vi "Chart_Formula_Manual_Incremental.vi"(7 "error in (no error)":errorcluster, 9 "Max Voltage":dbl, 10 "Min Voltage":dbl) -> ()   [LabVIEW 2020]
uses:
  Global 1.vi
panel:
  out "INDEX TI - 5th":i32
  out "ADDER TI - 5th":dbl
  out "INDEX TI - 4th":i32
  out "ADDER TI - 4th":dbl
  out "INDEX TI - 3rd":i32
  out "ADDER TI - 3rd":dbl
  out "INDEX TI - 2nd":i32
  out "ADDER TI - 2nd":dbl
  out "INDEX TI - 1st":i32
  out "size(s)":i32
  out "ADDER TI - 1st":dbl
  out "Array TI - 5th":dbl[](array[numeric])
  out "Array TI - 4th":dbl[](array[numeric])
  out "Array TI - 3rd":dbl[](array[numeric])
  out "Array TI - 2nd":dbl[](array[numeric])
  out "Array TI - 1st":dbl[](array[numeric])
  out "Chosen Max Voltage":dbl
  out "Chosen Min Voltage":dbl
  out "error out":errorcluster
  in  "CONFIRM CONDITION?":bool
  in  "Use 5th Threshold & Incremental ?":bool
  in  "Use 4th Threshold & Incremental ?":bool
  in  "Use 3rd Threshold & Incremental ?":bool
  in  "Use 2nd Threshold & Incremental ?":bool
  in  "Use 1st Threshold & Incremental ?":bool
  in  "Incremental 5":dbl
  in  "Threshold 5":dbl
  in  "Incremental 4":dbl
  in  "Threshold 4":dbl
  in  "Incremental 3":dbl
  in  "Threshold 3":dbl
  in  "Incremental 2":dbl
  in  "Threshold 2":dbl
  in  "Incremental 1":dbl
  in  "Threshold 1":dbl
  out "Array Result":dbl[](array[numeric])
  # "Manual Incremental : Increment at Threshold"
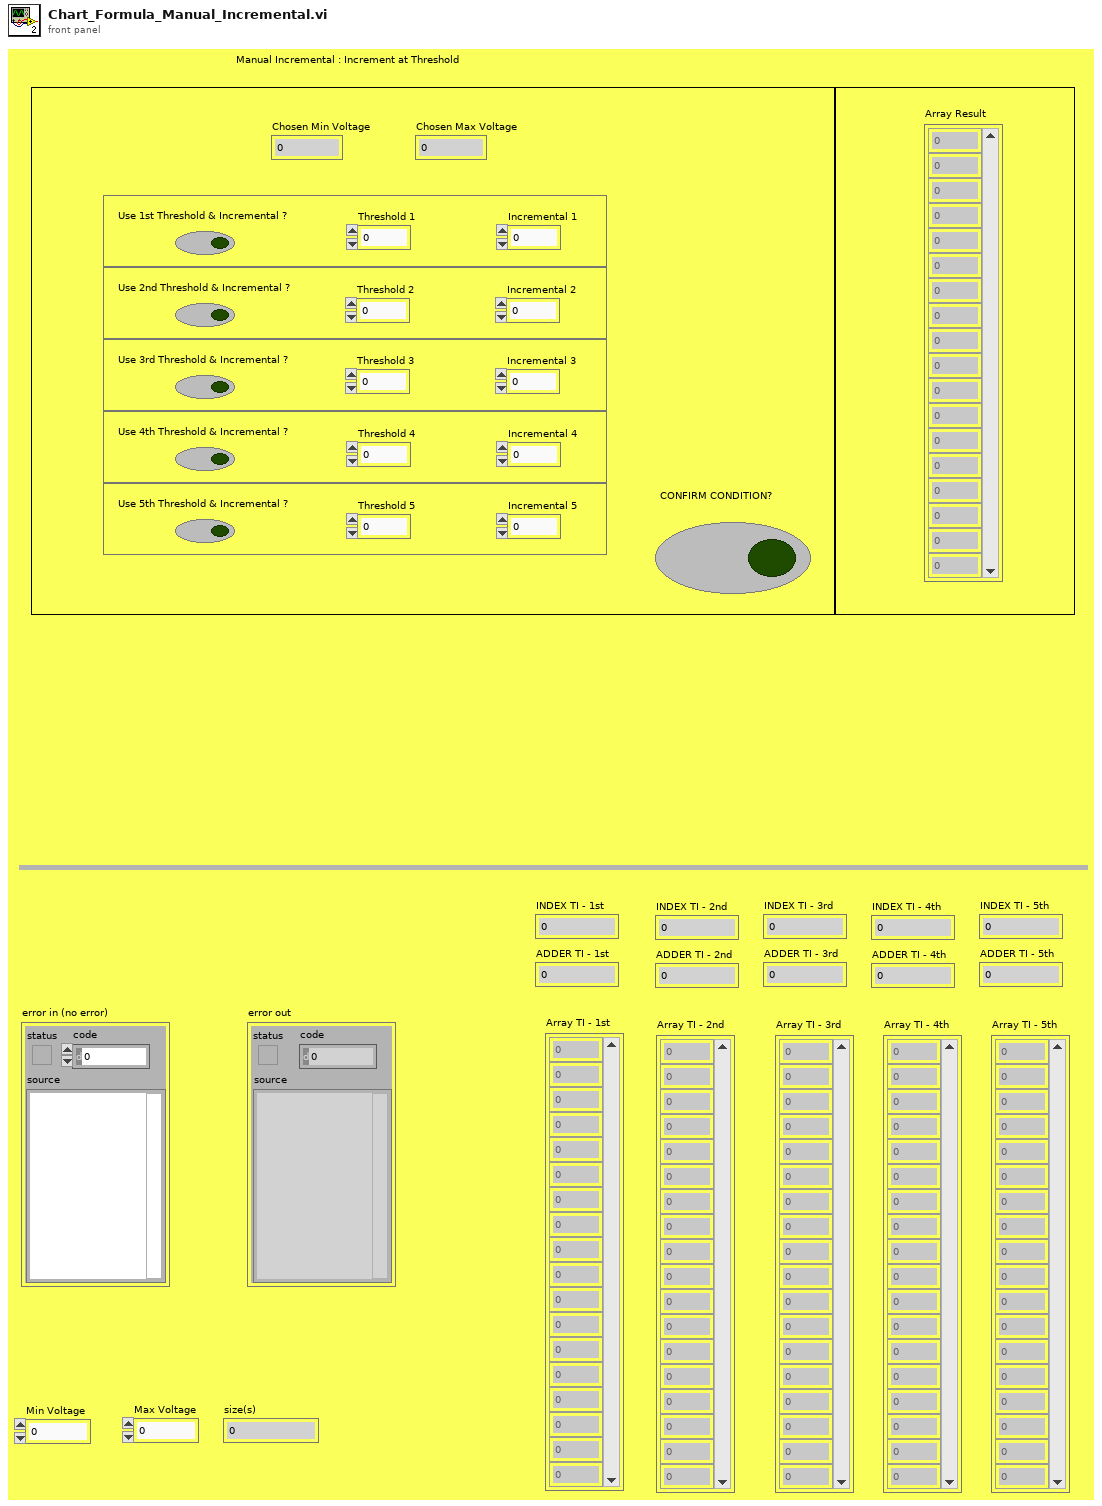
[diagram p1: front panel]
types:
  T1 = enum32{"Invalid", "Standard", "Closed", "Hidden", "Minimized", "Maximized"}
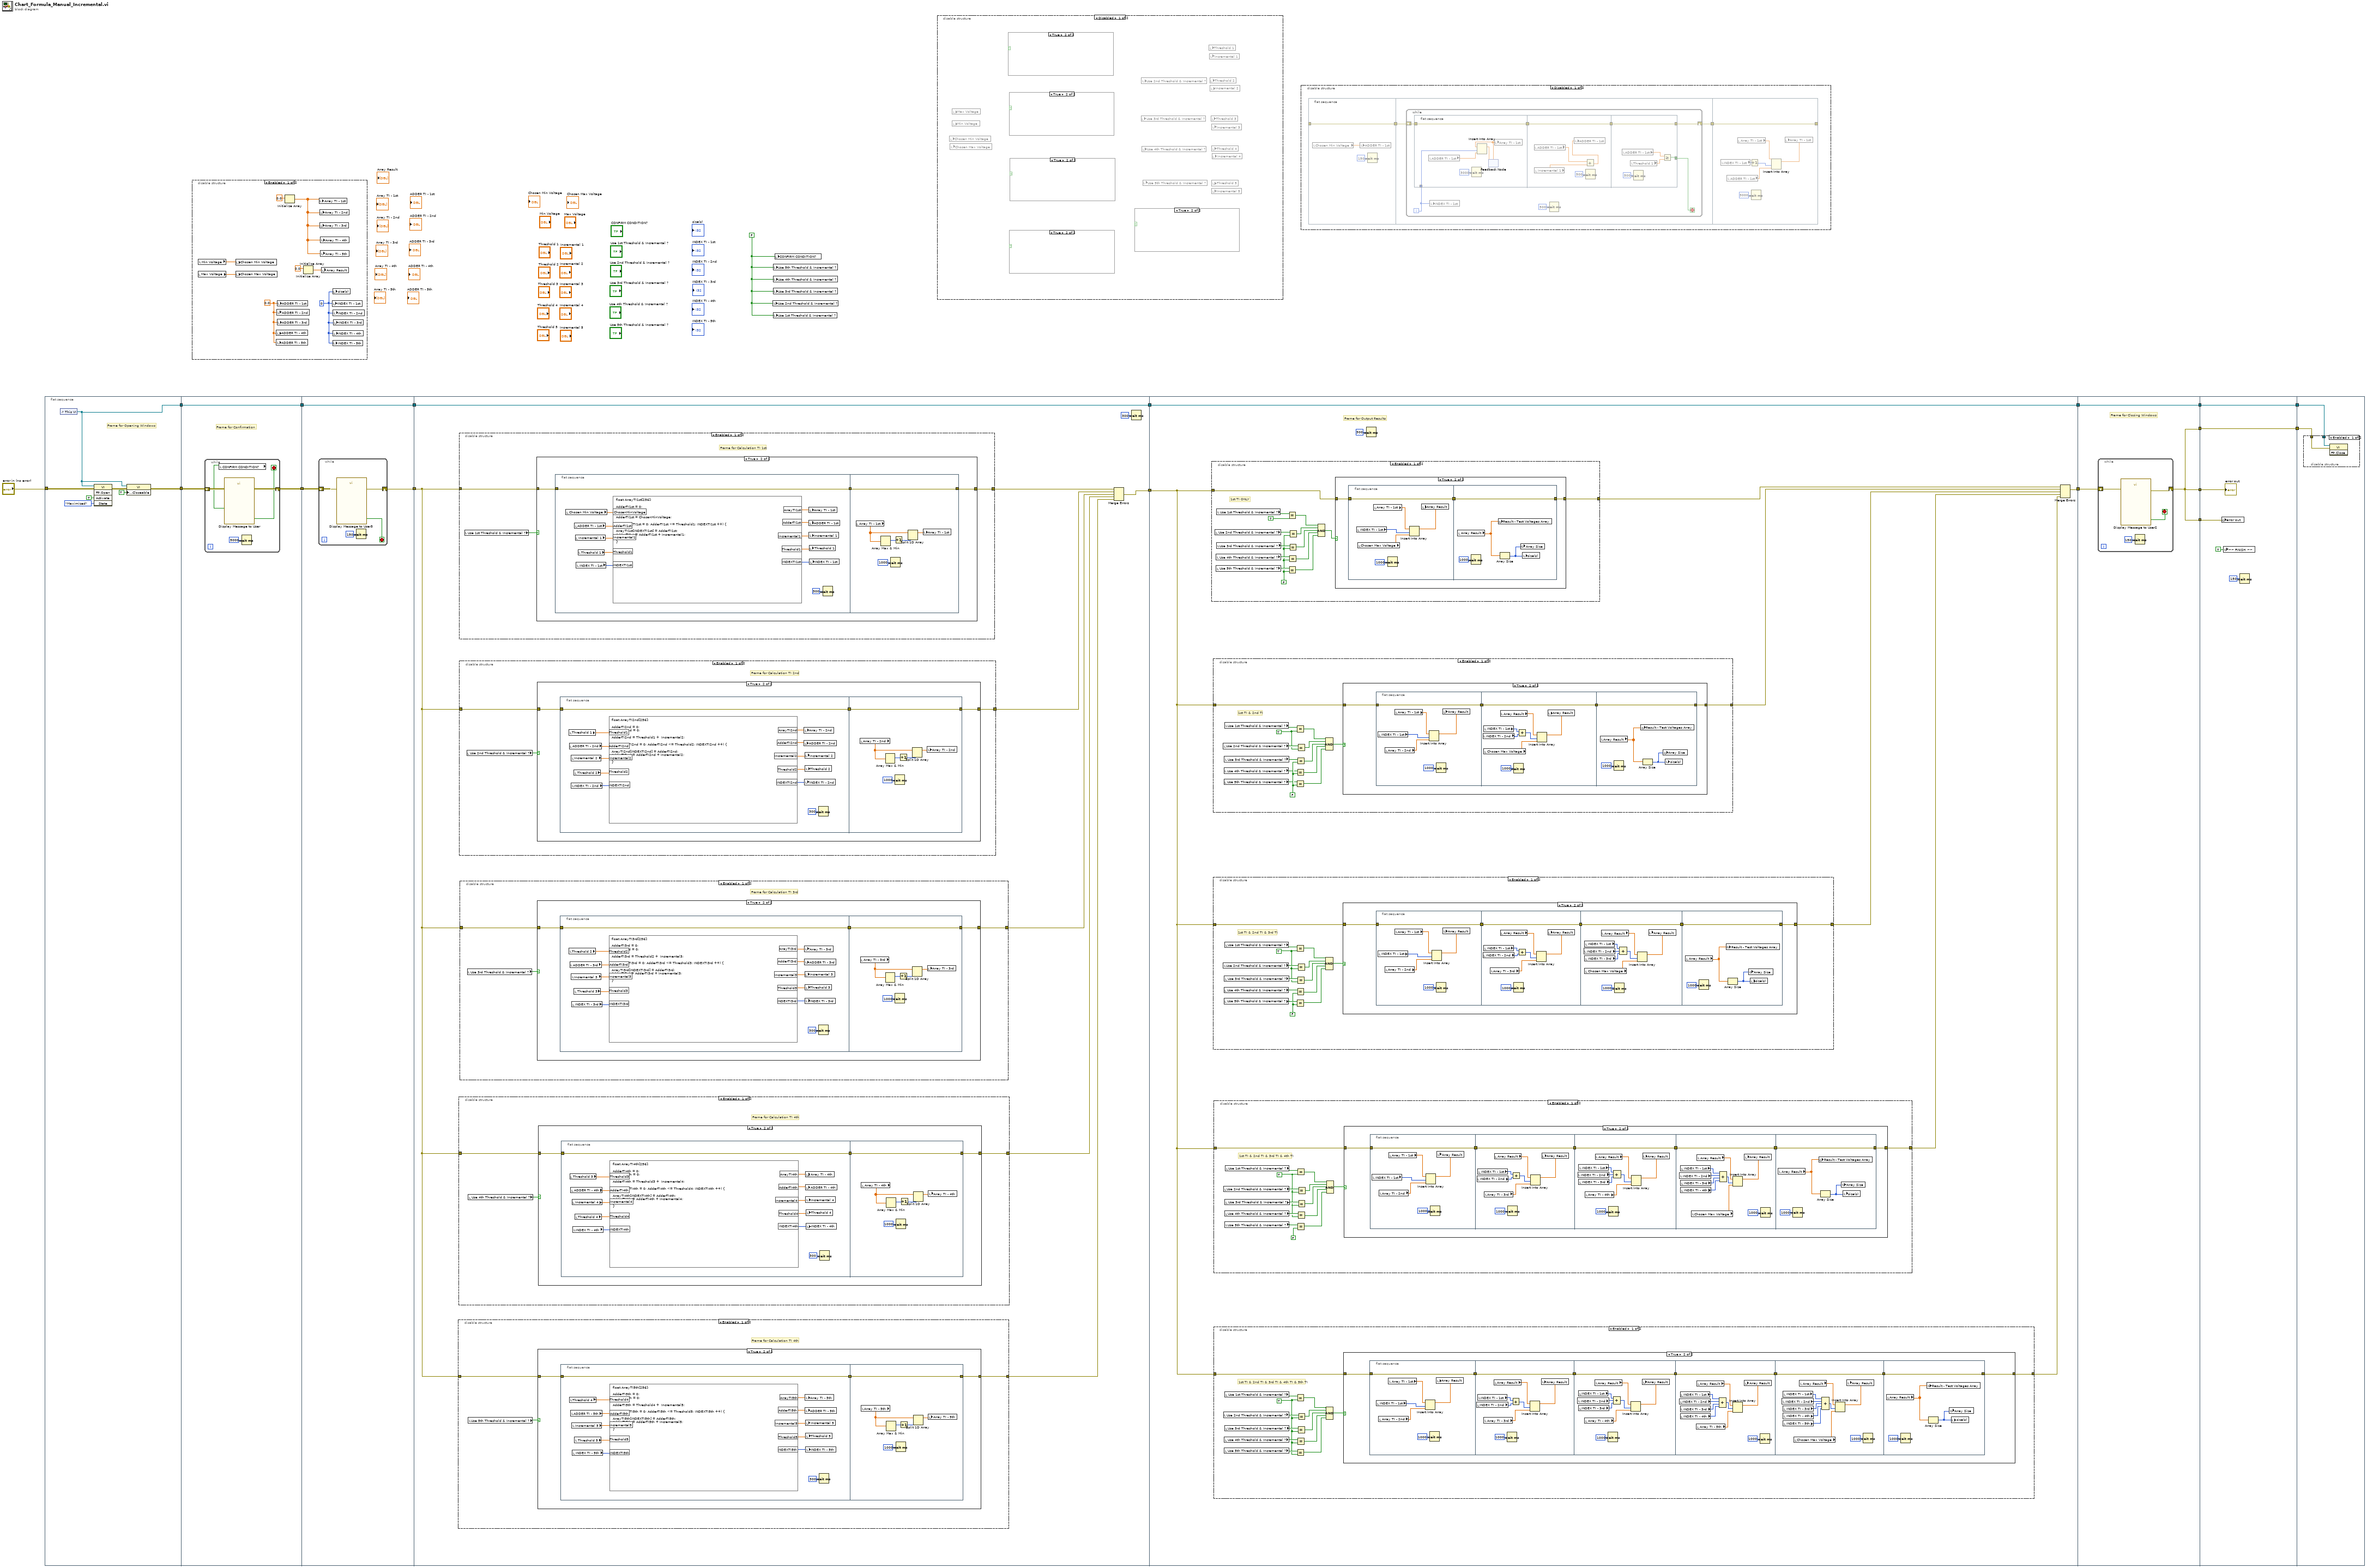
[diagram p0: block diagram]
diagram:
  w18 = FALSE
  n1 = flat-sequence {
    tunnel: "error in (no error)" -> [w21]
    tunnel: [w20] -> w1
    tunnel: [w19] -> w2
    tunnel: w2 -> [w27]
    tunnel: [w26] -> w8
    tunnel: w1 -> [w28]
    tunnel: [w28] -> w6
    tunnel: w8 -> [w35]
    tunnel: [w34] -> w7
    tunnel: w6 -> [w36]
    tunnel: [w36] -> w5
    tunnel: w7 -> [w42]
    tunnel: [w49] -> w4
    tunnel: w5 -> [w49]
    tunnel: [w46] -> w3
    tunnel: w4 -> [w183]
    tunnel: [w183] -> w16
    tunnel: [w181] -> w15
    tunnel: w3 -> [w176]
    tunnel: w16 -> [w429]
    tunnel: w15 -> [w430]
    tunnel: [w429] -> w14
    tunnel: [w428] -> w13
    tunnel: [w428] -> w12
    tunnel: [w428] -> w11
    tunnel: w14 -> [w436]
    tunnel: w13 -> [w435]
    tunnel: w12 -> [w439]
    tunnel: w11 -> [w438]
    tunnel: [w436] -> w10
    tunnel: [w435] -> w9
    tunnel: w10 -> [w442]
    tunnel: w9 -> [w441]
    frame #0 {
      # "Frame for Opening Windows"
      n2 = control-ref of="This VI"() -> (w20:refnum<vi>)
      n3 = invoke class="VI" method="FP.Open"(reference=w20, error in=w21, "Activate"=TRUE ("Activate?"), "State"=T1."Maximized") -> (error out=w22:errorcluster)  [unwired: 1 in, 4 out]
      n4 = property class="VI"(reference=w20, error in=w22, "Front Panel.Closeable"=TRUE ("Front Panel Window:Closeable")) -> (error out=w19:errorcluster)  [unwired: 1 out]
    }
    frame #1 {
      # "Frame for Confirmation"
      n5 = while {
        shift-right: [w29] -> w26
        shift-left: w27 -> [w30]
        stop <- w31 stop-if-true
        n6 = local read "CONFIRM CONDITION?"() -> (w32:bool)
        n7 = call "Display Message to User"("error in (no error)"=w30, "Enable"=w32) -> ("error out"=w29:errorcluster, "YES"=w31:bool)  [unwired: 8 in]
        n8 = Wait (ms)(milliseconds to wait=u32 5000) -> ()  [unwired: 1 out]
      }
    }
    frame #2 {
      n9 = while {
        shift-right: [w38] -> w34
        shift-left: w35 -> [w39]
        stop <- w40 stop-if-true
        n10 = call "Display Message to User3"("error in (no error)"=w39) -> ("error out"=w38:errorcluster, "OK"=w40:bool)  [unwired: 9 in]
        n11 = Wait (ms)(milliseconds to wait=u32 150) -> ()  [unwired: 1 out]
      }
    }
    frame #3 {
      n12 = disable-structure shown="Enabled" {
        disable-tunnel: w42 -> [w51 _]
        disable-tunnel: [w50 _] -> w41
        frame Enabled {
          # "Frame for Calculation TI 4th"
          n13 = local read "Use 5th Threshold & Incremental ?"() -> (w52:bool)
          n14 = case shown="True" w52 {
            tunnel: w51 -> [w53 w56]
            tunnel: [w53 w55] -> w50
            frame False {
            }
            frame True {
              n15 = flat-sequence {
                tunnel: w56 -> [w57]
                tunnel: [w57] -> w54
                tunnel: [w74] -> w55
                tunnel: w54 -> [w74]
                frame #0 {
                  n16 = local read "Threshold 4"() -> (w58:dbl)
                  n17 = local read "ADDER TI - 5th"() -> (w59:dbl)
                  n18 = local read "Incremental 5"() -> (w60:dbl)
                  n19 = local read "INDEX TI - 5th"() -> (w62:i32)
                  n20 = local read "Threshold 5"() -> (w61:dbl)
                  n21 = formula code="float ArrayTI5th[256];\n\nAdderTI5th = 0;\nINDEXTI5th = 0;\n\nAdderTI5th = Threshold4 +  Incremental5;\n\nfor (INDEXTI5th = 0; AdderTI5th <= Threshold5; INDEXTI5th ++) {\n\nArrayTI5th[INDEXTI5th] = AdderTI5th;\nAdderTI5th = AdderTI5th + Incremental5;\n\n}"("Threshold4"=w58, "AdderTI5th"=w59, "Incremental5"=w60, "Threshold5"=w61, "INDEXTI5th"=w62) -> ("ArrayTI5th"=w67:dbl[], "AdderTI5th"=w63:dbl, "Incremental5"=w64:dbl, "Threshold5"=w65:dbl, "INDEXTI5th"=w66:i32)
                  n22 = local write "Array TI - 5th"(w67) -> ()
                  n23 = local write "ADDER TI - 5th"(w63) -> ()
                  n24 = local write "Incremental 5"(w64) -> ()
                  n25 = local write "Threshold 5"(w65) -> ()
                  n26 = local write "INDEX TI - 5th"(w66) -> ()
                  n27 = Wait (ms)(milliseconds to wait=u32 300) -> ()  [unwired: 1 out]
                }
                frame #1 {
                  n28 = local read "Array TI - 5th"() -> (w71:dbl[])
                  n29 = Array Max & Min(array=w71) -> (max index (indices)=w73:i32)  [unwired: 3 out]
                  n30 = Wait (ms)(milliseconds to wait=u32 1000) -> ()  [unwired: 1 out]
                  n31 = Increment(x=w73) -> (x+1=w72:i32)
                  n32 = Split 1D Array(array=w71, index=w72) -> (first subarray=w70:dbl[])  [unwired: 1 out]
                  n33 = local write "Array TI - 5th"(w70) -> ()
                }
              }
            }
          }
        }
        frame Disabled {
        }
      }
      n34 = disable-structure shown="Enabled" {
        disable-tunnel: w42 -> [w126 _]
        disable-tunnel: [w125 _] -> w43
        frame Enabled {
          # "Frame for Calculation TI 4th"
          n35 = local read "Use 4th Threshold & Incremental ?"() -> (w127:bool)
          n36 = case shown="True" w127 {
            tunnel: w126 -> [w128 w131]
            tunnel: [w128 w130] -> w125
            frame False {
            }
            frame True {
              n37 = flat-sequence {
                tunnel: w131 -> [w132]
                tunnel: [w132] -> w129
                tunnel: [w149] -> w130
                tunnel: w129 -> [w149]
                frame #0 {
                  n38 = local read "Threshold 3"() -> (w133:dbl)
                  n39 = local read "ADDER TI - 4th"() -> (w134:dbl)
                  n40 = local read "Incremental 4"() -> (w135:dbl)
                  n41 = local read "INDEX TI - 4th"() -> (w137:i32)
                  n42 = local read "Threshold 4"() -> (w136:dbl)
                  n43 = formula code="float ArrayTI4th[256];\n\nAdderTI4th = 0;\nINDEXTI4th = 0;\n\nAdderTI4th = Threshold3 +  Incremental4;\n\nfor (INDEXTI4th = 0; AdderTI4th <= Threshold4; INDEXTI4th ++) {\n\nArrayTI4th[INDEXTI4th] = AdderTI4th;\nAdderTI4th = AdderTI4th + Incremental4;\n\n}"("Threshold3"=w133, "AdderTI4th"=w134, "Incremental4"=w135, "Threshold4"=w136, "INDEXTI4th"=w137) -> ("ArrayTI4th"=w142:dbl[], "AdderTI4th"=w138:dbl, "Incremental4"=w139:dbl, "Threshold4"=w140:dbl, "INDEXTI4th"=w141:i32)
                  n44 = local write "Array TI - 4th"(w142) -> ()
                  n45 = local write "ADDER TI - 4th"(w138) -> ()
                  n46 = local write "Incremental 4"(w139) -> ()
                  n47 = local write "Threshold 4"(w140) -> ()
                  n48 = local write "INDEX TI - 4th"(w141) -> ()
                  n49 = Wait (ms)(milliseconds to wait=u32 300) -> ()  [unwired: 1 out]
                }
                frame #1 {
                  n50 = local read "Array TI - 4th"() -> (w146:dbl[])
                  n51 = Array Max & Min(array=w146) -> (max index (indices)=w148:i32)  [unwired: 3 out]
                  n52 = Wait (ms)(milliseconds to wait=u32 1000) -> ()  [unwired: 1 out]
                  n53 = Increment(x=w148) -> (x+1=w147:i32)
                  n54 = Split 1D Array(array=w146, index=w147) -> (first subarray=w145:dbl[])  [unwired: 1 out]
                  n55 = local write "Array TI - 4th"(w145) -> ()
                }
              }
            }
          }
        }
        frame Disabled {
        }
      }
      n56 = disable-structure shown="Enabled" {
        disable-tunnel: [w101 _] -> w48
        disable-tunnel: w42 -> [w100 _]
        frame Enabled {
          # "Frame for Calculation TI 1st"
          n57 = local read "Use 1st Threshold & Incremental ?"() -> (w102:bool)
          n58 = case shown="True" w102 {
            tunnel: w100 -> [w103 w106]
            tunnel: [w103 w105] -> w101
            frame False {
            }
            frame True {
              n59 = flat-sequence {
                tunnel: w106 -> [w108]
                tunnel: [w108] -> w104
                tunnel: [w124] -> w105
                tunnel: w104 -> [w124]
                frame #0 {
                  n60 = local read "Chosen Min Voltage"() -> (w118:dbl)
                  n61 = local read "ADDER TI - 1st"() -> (w117:dbl)
                  n62 = local read "Incremental 1"() -> (w116:dbl)
                  n63 = local read "INDEX TI - 1st"() -> (w114:i32)
                  n64 = local read "Threshold 1"() -> (w115:dbl)
                  n65 = formula code="float ArrayTI1st[256];\n\nAdderTI1st = 0;\nINDEXTI1st = 0;\n\nAdderTI1st = ChosenMinVoltage;\n\nfor (INDEXTI1st = 0; AdderTI1st <= Threshold1; INDEXTI1st ++) {\n\nArrayTI1st[INDEXTI1st] = AdderTI1st;\nAdderTI1st = AdderTI1st + Incremental1;\n\n}"("ChosenMinVoltage"=w118, "AdderTI1st"=w117, "Incremental1"=w116, "Threshold1"=w115, "INDEXTI1st"=w114) -> ("ArrayTI1st"=w109:dbl[], "AdderTI1st"=w113:dbl, "Incremental1"=w112:dbl, "Threshold1"=w111:dbl, "INDEXTI1st"=w110:i32)
                  n66 = local write "Array TI - 1st"(w109) -> ()
                  n67 = local write "ADDER TI - 1st"(w113) -> ()
                  n68 = local write "Incremental 1"(w112) -> ()
                  n69 = local write "Threshold 1"(w111) -> ()
                  n70 = local write "INDEX TI - 1st"(w110) -> ()
                  n71 = Wait (ms)(milliseconds to wait=u32 300) -> ()  [unwired: 1 out]
                }
                frame #1 {
                  n72 = local read "Array TI - 1st"() -> (w121:dbl[])
                  n73 = Array Max & Min(array=w121) -> (max index (indices)=w123:i32)  [unwired: 3 out]
                  n74 = Wait (ms)(milliseconds to wait=u32 1000) -> ()  [unwired: 1 out]
                  n75 = Increment(x=w123) -> (x+1=w122:i32)
                  n76 = Split 1D Array(array=w121, index=w122) -> (first subarray=w120:dbl[])  [unwired: 1 out]
                  n77 = local write "Array TI - 1st"(w120) -> ()
                }
              }
            }
          }
        }
        frame Disabled {
        }
      }
      n78 = disable-structure shown="Enabled" {
        disable-tunnel: [w76 _] -> w47
        disable-tunnel: w42 -> [w75 _]
        frame Enabled {
          # "Frame for Calculation TI 2nd"
          n79 = local read "Use 2nd Threshold & Incremental ?"() -> (w77:bool)
          n80 = case shown="True" w77 {
            tunnel: w75 -> [w78 w81]
            tunnel: [w78 w80] -> w76
            frame False {
            }
            frame True {
              n81 = flat-sequence {
                tunnel: w81 -> [w82]
                tunnel: [w82] -> w79
                tunnel: [w99] -> w80
                tunnel: w79 -> [w99]
                frame #0 {
                  n82 = local read "Threshold 1"() -> (w83:dbl)
                  n83 = local read "ADDER TI - 2nd"() -> (w84:dbl)
                  n84 = local read "Incremental 2"() -> (w85:dbl)
                  n85 = local read "INDEX TI - 2nd"() -> (w87:i32)
                  n86 = local read "Threshold 2"() -> (w86:dbl)
                  n87 = formula code="float ArrayTI2nd[256];\n\nAdderTI2nd = 0;\nINDEXTI2nd = 0;\n\nAdderTI2nd = Threshold1 +  Incremental2;\n\nfor (INDEXTI2nd = 0; AdderTI2nd <= Threshold2; INDEXTI2nd ++) {\n\nArrayTI2nd[INDEXTI2nd] = AdderTI2nd;\nAdderTI2nd = AdderTI2nd + Incremental2;\n\n}"("Threshold1"=w83, "AdderTI2nd"=w84, "Incremental2"=w85, "Threshold2"=w86, "INDEXTI2nd"=w87) -> ("ArrayTI2nd"=w92:dbl[], "AdderTI2nd"=w88:dbl, "Incremental2"=w89:dbl, "Threshold2"=w90:dbl, "INDEXTI2nd"=w91:i32)
                  n88 = local write "ADDER TI - 2nd"(w88) -> ()
                  n89 = local write "Array TI - 2nd"(w92) -> ()
                  n90 = local write "INDEX TI - 2nd"(w91) -> ()
                  n91 = local write "Incremental 2"(w89) -> ()
                  n92 = local write "Threshold 2"(w90) -> ()
                  n93 = Wait (ms)(milliseconds to wait=u32 300) -> ()  [unwired: 1 out]
                }
                frame #1 {
                  n94 = local read "Array TI - 2nd"() -> (w96:dbl[])
                  n95 = Array Max & Min(array=w96) -> (max index (indices)=w98:i32)  [unwired: 3 out]
                  n96 = Wait (ms)(milliseconds to wait=u32 1000) -> ()  [unwired: 1 out]
                  n97 = Increment(x=w98) -> (x+1=w97:i32)
                  n98 = Split 1D Array(array=w96, index=w97) -> (first subarray=w95:dbl[])  [unwired: 1 out]
                  n99 = local write "Array TI - 2nd"(w95) -> ()
                }
              }
            }
          }
        }
        frame Disabled {
        }
      }
      n100 = disable-structure shown="Enabled" {
        disable-tunnel: w42 -> [w151 _]
        disable-tunnel: [w150 _] -> w44
        frame Enabled {
          # "Frame for Calculation TI 3rd"
          n101 = local read "Use 3rd Threshold & Incremental ?"() -> (w152:bool)
          n102 = case shown="True" w152 {
            tunnel: w151 -> [w153 w156]
            tunnel: [w153 w155] -> w150
            frame False {
            }
            frame True {
              n103 = flat-sequence {
                tunnel: w156 -> [w157]
                tunnel: [w157] -> w154
                tunnel: [w174] -> w155
                tunnel: w154 -> [w174]
                frame #0 {
                  n104 = local read "Threshold 2"() -> (w158:dbl)
                  n105 = local read "ADDER TI - 3rd"() -> (w159:dbl)
                  n106 = local read "Incremental 3"() -> (w160:dbl)
                  n107 = local read "INDEX TI - 3rd"() -> (w162:i32)
                  n108 = local read "Threshold 3"() -> (w161:dbl)
                  n109 = formula code="float ArrayTI3rd[256];\n\nAdderTI3rd = 0;\nINDEXTI3rd = 0;\n\nAdderTI3rd = Threshold2 +  Incremental3;\n\nfor (INDEXTI3rd = 0; AdderTI3rd <= Threshold3; INDEXTI3rd ++) {\n\nArrayTI3rd[INDEXTI3rd] = AdderTI3rd;\nAdderTI3rd = AdderTI3rd + Incremental3;\n\n}"("Threshold2"=w158, "AdderTI3rd"=w159, "Incremental3"=w160, "Threshold3"=w161, "INDEXTI3rd"=w162) -> ("ArrayTI3rd"=w167:dbl[], "AdderTI3rd"=w163:dbl, "Incremental3"=w164:dbl, "Threshold3"=w165:dbl, "INDEXTI3rd"=w166:i32)
                  n110 = local write "Array TI - 3rd"(w167) -> ()
                  n111 = local write "ADDER TI - 3rd"(w163) -> ()
                  n112 = local write "Incremental 3"(w164) -> ()
                  n113 = local write "Threshold 3"(w165) -> ()
                  n114 = local write "INDEX TI - 3rd"(w166) -> ()
                  n115 = Wait (ms)(milliseconds to wait=u32 300) -> ()  [unwired: 1 out]
                }
                frame #1 {
                  n116 = local read "Array TI - 3rd"() -> (w171:dbl[])
                  n117 = Array Max & Min(array=w171) -> (max index (indices)=w173:i32)  [unwired: 3 out]
                  n118 = Wait (ms)(milliseconds to wait=u32 1000) -> ()  [unwired: 1 out]
                  n119 = Increment(x=w173) -> (x+1=w172:i32)
                  n120 = Split 1D Array(array=w171, index=w172) -> (first subarray=w170:dbl[])  [unwired: 1 out]
                  n121 = local write "Array TI - 3rd"(w170) -> ()
                }
              }
            }
          }
        }
        frame Disabled {
        }
      }
      n122 = Merge Errors(w48, w47, w44, w43, w41) -> (w46:errorcluster)
      n123 = Wait (ms)(milliseconds to wait=u32 300) -> ()  [unwired: 1 out]
    }
    frame #4 {
      # "Frame for Output Results"
      n124 = disable-structure shown="Enabled" {
        disable-tunnel: [w352 _] -> w180
        disable-tunnel: w176 -> [w351 _]
        frame Enabled {
          w359 = FALSE
          # "1st TI ONLY"
          n125 = local read "Use 2nd Threshold & Incremental ?"() -> (w363:bool)
          n126 = local read "Use 4th Threshold & Incremental ?"() -> (w361:bool)
          n127 = local read "Use 5th Threshold & Incremental ?"() -> (w360:bool)
          n128 = local read "Use 3rd Threshold & Incremental ?"() -> (w362:bool)
          n129 = local read "Use 1st Threshold & Incremental ?"() -> (w365:bool)
          n130 = Equal?(x=w365, y=TRUE) -> (x = y?=w358:bool)
          n131 = Equal?(x=w360, y=w359) -> (x = y?=w354:bool)
          n132 = Equal?(x=w361, y=w359) -> (x = y?=w355:bool)
          n133 = Equal?(x=w362, y=w359) -> (x = y?=w356:bool)
          n134 = Equal?(x=w363, y=w359) -> (x = y?=w357:bool)
          n135 = Compound Arithmetic op=AND(w358, w357, w356, w355, w354) -> (w353:bool)
          n136 = case shown="True" w353 {
            tunnel: w351 -> [w366 w369]
            tunnel: [w366 w368] -> w352
            frame False {
            }
            frame True {
              n137 = flat-sequence {
                tunnel: w369 -> [w375]
                tunnel: [w375] -> w367
                tunnel: [w376] -> w368
                tunnel: w367 -> [w376]
                frame #0 {
                  n138 = local read "INDEX TI - 1st"() -> (w371:i32)
                  n139 = local read "Chosen Max Voltage"() -> (w374:dbl)
                  n140 = local read "Array TI - 1st"() -> (w372:dbl[])
                  n141 = Wait (ms)(milliseconds to wait=u32 1000) -> ()  [unwired: 1 out]
                  n142 = Insert Into Array(array=w372, index=w371, new element=w374) -> (w373:dbl[])
                  n143 = local write "Array Result"(w373) -> ()
                }
                frame #1 {
                  n144 = local read "Array Result"() -> (w378:dbl[])
                  n145 = Wait (ms)(milliseconds to wait=u32 1000) -> ()  [unwired: 1 out]
                  n146 = global write "Global 1.vi" "Result - Test Voltages Array"(w378) -> ()
                  n147 = Array Size(array=w378) -> (size(s)=w379:i32)
                  n148 = global write "Global 1.vi" "Array Size"(w379) -> ()
                  n149 = local write "size(s)"(w379) -> ()
                }
              }
            }
          }
        }
        frame Disabled {
        }
      }
      n150 = disable-structure shown="Enabled" {
        disable-tunnel: [w314 _] -> w179
        disable-tunnel: w176 -> [w313 _]
        frame Enabled {
          w322 = FALSE
          w316 = TRUE ("y")
          # "1st TI & 2nd TI"
          n151 = local read "Use 2nd Threshold & Incremental ?"() -> (w318:bool)
          n152 = local read "Use 4th Threshold & Incremental ?"() -> (w320:bool)
          n153 = local read "Use 5th Threshold & Incremental ?"() -> (w321:bool)
          n154 = local read "Use 3rd Threshold & Incremental ?"() -> (w319:bool)
          n155 = local read "Use 1st Threshold & Incremental ?"() -> (w317:bool)
          n156 = Equal?(x=w317, y=w316) -> (x = y?=w323:bool)
          n157 = Equal?(x=w321, y=w322) -> (x = y?=w327:bool)
          n158 = Equal?(x=w320, y=w322) -> (x = y?=w326:bool)
          n159 = Equal?(x=w319, y=w322) -> (x = y?=w325:bool)
          n160 = Equal?(x=w318, y=w316) -> (x = y?=w324:bool)
          n161 = Compound Arithmetic op=AND(w323, w324, w325, w326, w327) -> (w315:bool)
          n162 = case shown="True" w315 {
            tunnel: w313 -> [w328 w332]
            tunnel: [w328 w331] -> w314
            frame False {
            }
            frame True {
              n163 = flat-sequence {
                tunnel: w332 -> [w338]
                tunnel: [w338] -> w329
                tunnel: [w346] -> w330
                tunnel: w329 -> [w346]
                tunnel: [w347] -> w331
                tunnel: w330 -> [w347]
                frame #0 {
                  n164 = local read "INDEX TI - 1st"() -> (w337:i32)
                  n165 = local read "Array TI - 2nd"() -> (w334:dbl[])
                  n166 = local read "Array TI - 1st"() -> (w336:dbl[])
                  n167 = Insert Into Array(array=w336, index=w337, new element=w334) -> (w335:dbl[])
                  n168 = Wait (ms)(milliseconds to wait=u32 1000) -> ()  [unwired: 1 out]
                  n169 = local write "Array Result"(w335) -> ()
                }
                frame #1 {
                  n170 = local read "INDEX TI - 2nd"() -> (w340:i32)
                  n171 = local read "INDEX TI - 1st"() -> (w341:i32)
                  n172 = local read "Chosen Max Voltage"() -> (w345:dbl)
                  n173 = local read "Array Result"() -> (w343:dbl[])
                  n174 = Wait (ms)(milliseconds to wait=u32 1000) -> ()  [unwired: 1 out]
                  n175 = Add(x=w341, y=w340) -> (x+y=w339:i32)
                  n176 = Insert Into Array(array=w343, index=w339, new element=w345) -> (w344:dbl[])
                  n177 = local write "Array Result"(w344) -> ()
                }
                frame #2 {
                  n178 = local read "Array Result"() -> (w349:dbl[])
                  n179 = Wait (ms)(milliseconds to wait=u32 1000) -> ()  [unwired: 1 out]
                  n180 = global write "Global 1.vi" "Result - Test Voltages Array"(w349) -> ()
                  n181 = Array Size(array=w349) -> (size(s)=w350:i32)
                  n182 = global write "Global 1.vi" "Array Size"(w350) -> ()
                  n183 = local write "size(s)"(w350) -> ()
                }
              }
            }
          }
        }
        frame Disabled {
        }
      }
      n184 = disable-structure shown="Enabled" {
        disable-tunnel: [w381 _] -> w178
        disable-tunnel: w176 -> [w380 _]
        frame Enabled {
          w388 = FALSE
          w382 = TRUE ("y")
          # "1st TI & 2nd TI & 3rd TI"
          n185 = local read "Use 2nd Threshold & Incremental ?"() -> (w392:bool)
          n186 = local read "Use 4th Threshold & Incremental ?"() -> (w390:bool)
          n187 = local read "Use 5th Threshold & Incremental ?"() -> (w389:bool)
          n188 = local read "Use 3rd Threshold & Incremental ?"() -> (w391:bool)
          n189 = local read "Use 1st Threshold & Incremental ?"() -> (w393:bool)
          n190 = Equal?(x=w393, y=w382) -> (x = y?=w387:bool)
          n191 = Equal?(x=w389, y=w388) -> (x = y?=w383:bool)
          n192 = Equal?(x=w390, y=w388) -> (x = y?=w384:bool)
          n193 = Equal?(x=w391, y=w382) -> (x = y?=w385:bool)
          n194 = Equal?(x=w392, y=w382) -> (x = y?=w386:bool)
          n195 = Compound Arithmetic op=AND(w387, w386, w385, w384, w383) -> (w394:bool)
          n196 = case shown="True" w394 {
            tunnel: w380 -> [w395 w400]
            tunnel: [w395 w399] -> w381
            frame False {
            }
            frame True {
              n197 = flat-sequence {
                tunnel: w400 -> [w406]
                tunnel: [w406] -> w398
                tunnel: [w414] -> w397
                tunnel: w398 -> [w414]
                tunnel: w397 -> [w423]
                tunnel: [w423] -> w396
                tunnel: [w424] -> w399
                tunnel: w396 -> [w424]
                frame #0 {
                  n198 = local read "INDEX TI - 1st"() -> (w405:i32)
                  n199 = local read "Array TI - 2nd"() -> (w402:dbl[])
                  n200 = local read "Array TI - 1st"() -> (w404:dbl[])
                  n201 = Insert Into Array(array=w404, index=w405, new element=w402) -> (w403:dbl[])
                  n202 = Wait (ms)(milliseconds to wait=u32 1000) -> ()  [unwired: 1 out]
                  n203 = local write "Array Result"(w403) -> ()
                }
                frame #1 {
                  n204 = local read "INDEX TI - 2nd"() -> (w408:i32)
                  n205 = local read "INDEX TI - 1st"() -> (w409:i32)
                  n206 = local read "Array TI - 3rd"() -> (w413:dbl[])
                  n207 = local read "Array Result"() -> (w411:dbl[])
                  n208 = Wait (ms)(milliseconds to wait=u32 1000) -> ()  [unwired: 1 out]
                  n209 = Add(x=w409, y=w408) -> (x+y=w407:i32)
                  n210 = Insert Into Array(array=w411, index=w407, new element=w413) -> (w412:dbl[])
                  n211 = local write "Array Result"(w412) -> ()
                }
                frame #2 {
                  n212 = local read "INDEX TI - 2nd"() -> (w417:i32)
                  n213 = local read "INDEX TI - 1st"() -> (w418:i32)
                  n214 = local read "INDEX TI - 3rd"() -> (w416:i32)
                  n215 = local read "Chosen Max Voltage"() -> (w419:dbl)
                  n216 = local read "Array Result"() -> (w421:dbl[])
                  n217 = Wait (ms)(milliseconds to wait=u32 1000) -> ()  [unwired: 1 out]
                  n218 = Compound Arithmetic op=ADD(w418, w417, w416) -> (w415:i32)
                  n219 = Insert Into Array(array=w421, index=w415, new element=w419) -> (w420:dbl[])
                  n220 = local write "Array Result"(w420) -> ()
                }
                frame #3 {
                  n221 = local read "Array Result"() -> (w426:dbl[])
                  n222 = Wait (ms)(milliseconds to wait=u32 1000) -> ()  [unwired: 1 out]
                  n223 = global write "Global 1.vi" "Result - Test Voltages Array"(w426) -> ()
                  n224 = Array Size(array=w426) -> (size(s)=w427:i32)
                  n225 = global write "Global 1.vi" "Array Size"(w427) -> ()
                  n226 = local write "size(s)"(w427) -> ()
                }
              }
            }
          }
        }
        frame Disabled {
        }
      }
      n227 = disable-structure shown="Enabled" {
        disable-tunnel: [w186 _] -> w175
        disable-tunnel: w176 -> [w185 _]
        frame Enabled {
          w184 = TRUE ("y")
          # "1st TI & 2nd TI & 3rd TI & 4th TI & 5th TI"
          n228 = local read "Use 2nd Threshold & Incremental ?"() -> (w195:bool)
          n229 = local read "Use 4th Threshold & Incremental ?"() -> (w193:bool)
          n230 = local read "Use 5th Threshold & Incremental ?"() -> (w192:bool)
          n231 = local read "Use 3rd Threshold & Incremental ?"() -> (w194:bool)
          n232 = local read "Use 1st Threshold & Incremental ?"() -> (w196:bool)
          n233 = Equal?(x=w196, y=w184) -> (x = y?=w191:bool)
          n234 = Equal?(x=w192, y=w184) -> (x = y?=w187:bool)
          n235 = Equal?(x=w193, y=w184) -> (x = y?=w188:bool)
          n236 = Equal?(x=w194, y=w184) -> (x = y?=w189:bool)
          n237 = Equal?(x=w195, y=w184) -> (x = y?=w190:bool)
          n238 = Compound Arithmetic op=AND(w191, w190, w189, w188, w187) -> (w197:bool)
          n239 = case shown="True" w197 {
            tunnel: w185 -> [w198 w205]
            tunnel: [w198 w204] -> w186
            frame False {
            }
            frame True {
              n240 = flat-sequence {
                tunnel: w205 -> [w211]
                tunnel: [w211] -> w203
                tunnel: [w219] -> w202
                tunnel: w203 -> [w219]
                tunnel: w202 -> [w228]
                tunnel: [w228] -> w201
                tunnel: w201 -> [w238]
                tunnel: [w238] -> w200
                tunnel: w200 -> [w249]
                tunnel: [w249] -> w199
                tunnel: [w250] -> w204
                tunnel: w199 -> [w250]
                frame #0 {
                  n241 = local read "INDEX TI - 1st"() -> (w210:i32)
                  n242 = local read "Array TI - 2nd"() -> (w207:dbl[])
                  n243 = local read "Array TI - 1st"() -> (w209:dbl[])
                  n244 = Insert Into Array(array=w209, index=w210, new element=w207) -> (w208:dbl[])
                  n245 = Wait (ms)(milliseconds to wait=u32 1000) -> ()  [unwired: 1 out]
                  n246 = local write "Array Result"(w208) -> ()
                }
                frame #1 {
                  n247 = local read "INDEX TI - 2nd"() -> (w213:i32)
                  n248 = local read "INDEX TI - 1st"() -> (w214:i32)
                  n249 = local read "Array TI - 3rd"() -> (w218:dbl[])
                  n250 = local read "Array Result"() -> (w216:dbl[])
                  n251 = Wait (ms)(milliseconds to wait=u32 1000) -> ()  [unwired: 1 out]
                  n252 = Add(x=w214, y=w213) -> (x+y=w212:i32)
                  n253 = Insert Into Array(array=w216, index=w212, new element=w218) -> (w217:dbl[])
                  n254 = local write "Array Result"(w217) -> ()
                }
                frame #2 {
                  n255 = local read "INDEX TI - 2nd"() -> (w222:i32)
                  n256 = local read "INDEX TI - 1st"() -> (w223:i32)
                  n257 = local read "INDEX TI - 3rd"() -> (w221:i32)
                  n258 = local read "Array TI - 4th"() -> (w224:dbl[])
                  n259 = local read "Array Result"() -> (w226:dbl[])
                  n260 = Wait (ms)(milliseconds to wait=u32 1000) -> ()  [unwired: 1 out]
                  n261 = Compound Arithmetic op=ADD(w223, w222, w221) -> (w220:i32)
                  n262 = Insert Into Array(array=w226, index=w220, new element=w224) -> (w225:dbl[])
                  n263 = local write "Array Result"(w225) -> ()
                }
                frame #3 {
                  n264 = local read "INDEX TI - 2nd"() -> (w235:i32)
                  n265 = local read "INDEX TI - 1st"() -> (w234:i32)
                  n266 = local read "INDEX TI - 3rd"() -> (w236:i32)
                  n267 = local read "INDEX TI - 4th"() -> (w229:i32)
                  n268 = local read "Array TI - 5th"() -> (w233:dbl[])
                  n269 = local read "Array Result"() -> (w231:dbl[])
                  n270 = Compound Arithmetic op=ADD(w234, w235, w236, w229) -> (w237:i32)
                  n271 = Insert Into Array(array=w231, index=w237, new element=w233) -> (w232:dbl[])
                  n272 = local write "Array Result"(w232) -> ()
                  n273 = Wait (ms)(milliseconds to wait=u32 1000) -> ()  [unwired: 1 out]
                }
                frame #4 {
                  n274 = local read "INDEX TI - 2nd"() -> (w242:i32)
                  n275 = local read "INDEX TI - 1st"() -> (w243:i32)
                  n276 = local read "INDEX TI - 3rd"() -> (w241:i32)
                  n277 = local read "INDEX TI - 4th"() -> (w248:i32)
                  n278 = local read "INDEX TI - 5th"() -> (w239:i32)
                  n279 = local read "Chosen Max Voltage"() -> (w244:dbl)
                  n280 = local read "Array Result"() -> (w246:dbl[])
                  n281 = Compound Arithmetic op=ADD(w243, w242, w241, w248, w239) -> (w240:i32)
                  n282 = Insert Into Array(array=w246, index=w240, new element=w244) -> (w245:dbl[])
                  n283 = local write "Array Result"(w245) -> ()
                  n284 = Wait (ms)(milliseconds to wait=u32 1000) -> ()  [unwired: 1 out]
                }
                frame #5 {
                  n285 = local read "Array Result"() -> (w252:dbl[])
                  n286 = Wait (ms)(milliseconds to wait=u32 1000) -> ()  [unwired: 1 out]
                  n287 = global write "Global 1.vi" "Result - Test Voltages Array"(w252) -> ()
                  n288 = Array Size(array=w252) -> (size(s)=w253:i32)
                  n289 = global write "Global 1.vi" "Array Size"(w253) -> ()
                  n290 = local write "size(s)"(w253) -> ()
                }
              }
            }
          }
        }
        frame Disabled {
        }
      }
      n291 = disable-structure shown="Enabled" {
        disable-tunnel: [w256 _] -> w177
        disable-tunnel: w176 -> [w255 _]
        frame Enabled {
          w254 = TRUE ("y")
          # "1st TI & 2nd TI & 3rd TI & 4th TI"
          n292 = local read "Use 2nd Threshold & Incremental ?"() -> (w266:bool)
          n293 = local read "Use 4th Threshold & Incremental ?"() -> (w264:bool)
          n294 = local read "Use 5th Threshold & Incremental ?"() -> (w263:bool)
          n295 = local read "Use 3rd Threshold & Incremental ?"() -> (w265:bool)
          n296 = local read "Use 1st Threshold & Incremental ?"() -> (w267:bool)
          n297 = Equal?(x=w267, y=w254) -> (x = y?=w261:bool)
          n298 = Equal?(x=w263, y=FALSE) -> (x = y?=w257:bool)
          n299 = Equal?(x=w264, y=w254) -> (x = y?=w258:bool)
          n300 = Equal?(x=w265, y=w254) -> (x = y?=w259:bool)
          n301 = Equal?(x=w266, y=w254) -> (x = y?=w260:bool)
          n302 = Compound Arithmetic op=AND(w261, w260, w259, w258, w257) -> (w268:bool)
          n303 = case shown="True" w268 {
            tunnel: w255 -> [w269 w275]
            tunnel: [w269 w274] -> w256
            frame False {
            }
            frame True {
              n304 = flat-sequence {
                tunnel: w275 -> [w281]
                tunnel: [w281] -> w273
                tunnel: [w289] -> w272
                tunnel: w273 -> [w289]
                tunnel: w272 -> [w298]
                tunnel: [w298] -> w271
                tunnel: w271 -> [w308]
                tunnel: [w308] -> w270
                tunnel: [w309] -> w274
                tunnel: w270 -> [w309]
                frame #0 {
                  n305 = local read "INDEX TI - 1st"() -> (w280:i32)
                  n306 = local read "Array TI - 2nd"() -> (w277:dbl[])
                  n307 = local read "Array TI - 1st"() -> (w279:dbl[])
                  n308 = Insert Into Array(array=w279, index=w280, new element=w277) -> (w278:dbl[])
                  n309 = Wait (ms)(milliseconds to wait=u32 1000) -> ()  [unwired: 1 out]
                  n310 = local write "Array Result"(w278) -> ()
                }
                frame #1 {
                  n311 = local read "INDEX TI - 2nd"() -> (w283:i32)
                  n312 = local read "INDEX TI - 1st"() -> (w284:i32)
                  n313 = local read "Array TI - 3rd"() -> (w288:dbl[])
                  n314 = local read "Array Result"() -> (w286:dbl[])
                  n315 = Wait (ms)(milliseconds to wait=u32 1000) -> ()  [unwired: 1 out]
                  n316 = Add(x=w284, y=w283) -> (x+y=w282:i32)
                  n317 = Insert Into Array(array=w286, index=w282, new element=w288) -> (w287:dbl[])
                  n318 = local write "Array Result"(w287) -> ()
                }
                frame #2 {
                  n319 = local read "INDEX TI - 2nd"() -> (w292:i32)
                  n320 = local read "INDEX TI - 1st"() -> (w293:i32)
                  n321 = local read "INDEX TI - 3rd"() -> (w291:i32)
                  n322 = local read "Array TI - 4th"() -> (w294:dbl[])
                  n323 = local read "Array Result"() -> (w296:dbl[])
                  n324 = Wait (ms)(milliseconds to wait=u32 1000) -> ()  [unwired: 1 out]
                  n325 = Compound Arithmetic op=ADD(w293, w292, w291) -> (w290:i32)
                  n326 = Insert Into Array(array=w296, index=w290, new element=w294) -> (w295:dbl[])
                  n327 = local write "Array Result"(w295) -> ()
                }
                frame #3 {
                  n328 = local read "INDEX TI - 2nd"() -> (w305:i32)
                  n329 = local read "INDEX TI - 1st"() -> (w304:i32)
                  n330 = local read "INDEX TI - 3rd"() -> (w306:i32)
                  n331 = local read "INDEX TI - 4th"() -> (w299:i32)
                  n332 = local read "Chosen Max Voltage"() -> (w303:dbl)
                  n333 = local read "Array Result"() -> (w301:dbl[])
                  n334 = Compound Arithmetic op=ADD(w304, w305, w306, w299) -> (w307:i32)
                  n335 = Insert Into Array(array=w301, index=w307, new element=w303) -> (w302:dbl[])
                  n336 = local write "Array Result"(w302) -> ()
                  n337 = Wait (ms)(milliseconds to wait=u32 1000) -> ()  [unwired: 1 out]
                }
                frame #4 {
                  n338 = local read "Array Result"() -> (w311:dbl[])
                  n339 = Wait (ms)(milliseconds to wait=u32 1000) -> ()  [unwired: 1 out]
                  n340 = global write "Global 1.vi" "Result - Test Voltages Array"(w311) -> ()
                  n341 = Array Size(array=w311) -> (size(s)=w312:i32)
                  n342 = global write "Global 1.vi" "Array Size"(w312) -> ()
                  n343 = local write "size(s)"(w312) -> ()
                }
              }
            }
          }
        }
        frame Disabled {
        }
      }
      n344 = Wait (ms)(milliseconds to wait=u32 300) -> ()  [unwired: 1 out]
      n345 = Merge Errors(w180, w179, w178, w177, w175) -> (w181:errorcluster)
    }
    frame #5 {
      # "Frame for Closing Windows"
      n346 = while {
        shift-right: [w431] -> w428
        shift-left: w430 -> [w432]
        stop <- w433 stop-if-true
        n347 = call "Display Message to User2"("error in (no error)"=w432) -> ("error out"=w431:errorcluster, "OK"=w433:bool)  [unwired: 9 in]
        n348 = Wait (ms)(milliseconds to wait=u32 150) -> ()  [unwired: 1 out]
      }
    }
    frame #6 {
      n349 = global write "Global 1.vi" "error out"(w439) -> ()
      n350 = global write "Global 1.vi" "~~ FINISH ~~"(TRUE ("~~ FINISH ~~")) -> ()
      n351 = Wait (ms)(milliseconds to wait=u32 150) -> ()  [unwired: 1 out]
      "error out" <- w438
    }
    frame #7 {
      n352 = disable-structure shown="Enabled" {
        disable-tunnel: w442 -> [w444 _]
        disable-tunnel: w441 -> [w443 _]
        frame Enabled {
          n353 = invoke class="VI" method="FP.Close"(reference=w444, error in=w443) -> ()  [unwired: 1 in, 3 out]
        }
        frame Disabled {
        }
      }
    }
  }
  n354 = disable-structure shown="Enabled" {
    frame Enabled {
      w447 = 0 ("Index TI 1st")
      w448 = 0.0 ("ADDER T1 - 1st")
      n355 = local read "Max Voltage"() -> (w445:dbl)
      n356 = local read "Min Voltage"() -> (w446:dbl)
      n357 = local write "Chosen Min Voltage"(w446) -> ()
      n358 = local write "Chosen Max Voltage"(w445) -> ()
      n359 = local write "ADDER TI - 4th"(w448) -> ()
      n360 = local write "ADDER TI - 5th"(w448) -> ()
      n361 = local write "ADDER TI - 2nd"(w448) -> ()
      n362 = local write "ADDER TI - 1st"(w448) -> ()
      n363 = local write "ADDER TI - 3rd"(w448) -> ()
      n364 = Initialize Array(0.0 ("element")) -> (w452:dbl[])  [unwired: 1 in]
      n365 = Initialize Array(0.0 ("element")) -> ()  [unwired: 1 in, 1 out]
      n366 = Initialize Array(0.0 ("element")) -> (w451:dbl[])  [unwired: 1 in]
      n367 = local write "Array TI - 1st"(w452) -> ()
      n368 = local write "Array TI - 2nd"(w452) -> ()
      n369 = local write "Array TI - 3rd"(w452) -> ()
      n370 = local write "Array TI - 4th"(w452) -> ()
      n371 = local write "Array TI - 5th"(w452) -> ()
      n372 = local write "Array Result"(w451) -> ()
      n373 = local write "INDEX TI - 1st"(w447) -> ()
      n374 = local write "size(s)"(w447) -> ()
      n375 = local write "INDEX TI - 5th"(w447) -> ()
      n376 = local write "INDEX TI - 2nd"(w447) -> ()
      n377 = local write "INDEX TI - 4th"(w447) -> ()
      n378 = local write "INDEX TI - 3rd"(w447) -> ()
    }
    frame Disabled {
    }
  }
  n379 = local write "Use 2nd Threshold & Incremental ?"(w18) -> ()
  n380 = local write "Use 5th Threshold & Incremental ?"(w18) -> ()
  n381 = local write "Use 4th Threshold & Incremental ?"(w18) -> ()
  n382 = local write "Use 3rd Threshold & Incremental ?"(w18) -> ()
  n383 = local write "Use 1st Threshold & Incremental ?"(w18) -> ()
  n384 = local write "CONFIRM CONDITION?"(w18) -> ()
  n385 = disable-structure shown="Disabled" {
    frame Disabled {
      n386 = local read "Chosen Min Voltage"() -> ()  [unwired: 1 in]
      n387 = local read "Chosen Max Voltage"() -> ()  [unwired: 1 in]
      n388 = local read "Max Voltage"() -> ()  [unwired: 1 in]
      n389 = local read "Min Voltage"() -> ()  [unwired: 1 in]
      n390 = case shown="True" {
        selector: _ -> [_ _]
        frame False {
        }
        frame True {
        }
      }
      n391 = case shown="True" {
        selector: _ -> [_ _]
        frame False {
        }
        frame True {
        }
      }
      n392 = case shown="True" {
        selector: _ -> [_ _]
        frame False {
        }
        frame True {
        }
      }
      n393 = case shown="True" {
        selector: _ -> [_ _]
        frame False {
        }
        frame True {
        }
      }
      n394 = case shown="True" {
        selector: _ -> [_ _]
        frame False {
        }
        frame True {
        }
      }
      n395 = local read "Use 3rd Threshold & Incremental ?"() -> ()  [unwired: 1 in]
      n396 = local read "Use 2nd Threshold & Incremental ?"() -> ()  [unwired: 1 in]
      n397 = local read "Use 4th Threshold & Incremental ?"() -> ()  [unwired: 1 in]
      n398 = local read "Use 5th Threshold & Incremental ?"() -> ()  [unwired: 1 in]
      n399 = local read "Threshold 1"() -> ()  [unwired: 1 in]
      n400 = local read "Incremental 1"() -> ()  [unwired: 1 in]
      n401 = local read "Threshold 2"() -> ()  [unwired: 1 in]
      n402 = local read "Incremental 2"() -> ()  [unwired: 1 in]
      n403 = local read "Threshold 3"() -> ()  [unwired: 1 in]
      n404 = local read "Incremental 3"() -> ()  [unwired: 1 in]
      n405 = local read "Threshold 4"() -> ()  [unwired: 1 in]
      n406 = local read "Threshold 5"() -> ()  [unwired: 1 in]
      n407 = local read "Incremental 5"() -> ()  [unwired: 1 in]
      n408 = local read "Incremental 4"() -> ()  [unwired: 1 in]
    }
    frame Enabled {
    }
  }
  n409 = disable-structure shown="Disabled" {
    frame Disabled {
      n410 = flat-sequence {
        tunnel: _ -> [w458]
        tunnel: [w458] -> w455
        tunnel: w455 -> [w459]
        tunnel: [w460] -> w454
        tunnel: [w490] -> _
        tunnel: w454 -> [w490]
        frame #0 {
          n411 = local read "Chosen Min Voltage"() -> (w457:dbl)
          n412 = local write "ADDER TI - 1st"(w457) -> ()
          n413 = Wait (ms)(milliseconds to wait=u32 150) -> ()  [unwired: 1 out]
        }
        frame #1 {
          n414 = while {
            shift-right: [w463] -> w460
            shift-left: w459 -> [w466]
            i -> [w461]
            stop <- w467 stop-if-true
            n415 = flat-sequence {
              tunnel: w461 -> [w473]
              tunnel: w466 -> [w469]
              tunnel: [w469] -> w465
              tunnel: w465 -> [w475]
              tunnel: [w475] -> w464
              tunnel: [w482] -> w467
              tunnel: w464 -> [w480]
              tunnel: [w480] -> w463
              frame #0 {
                n416 = local read "ADDER TI - 1st"() -> (w470:dbl)
                n417 = Wait (ms)(milliseconds to wait=u32 3000) -> ()  [unwired: 1 out]
                n418 = feedback #1() -> (w471:dbl[])  [unwired: 1 in]
                n419 = Insert Into Array(array=w471, index=w473, new element=w470) -> (w472:dbl[])
                n420 = feedback-in #1(w472) -> ()
                n421 = local write "Array TI - 1st"(w471) -> ()
              }
              frame #1 {
                n422 = local read "ADDER TI - 1st"() -> (w477:dbl)
                n423 = local read "Incremental 1"() -> (w478:dbl)
                n424 = Add(x=w477, y=w478) -> (x+y=w476:dbl)
                n425 = local write "ADDER TI - 1st"(w476) -> ()
                n426 = Wait (ms)(milliseconds to wait=u32 500) -> ()  [unwired: 1 out]
              }
              frame #2 {
                n427 = local read "ADDER TI - 1st"() -> (w481:dbl)
                n428 = local read "Threshold 1"() -> (w483:dbl)
                n429 = Wait (ms)(milliseconds to wait=u32 500) -> ()  [unwired: 1 out]
                n430 = Greater Or Equal?(x=w481, y=w483) -> (x >= y?=w482:bool)
              }
            }
            n431 = local write "INDEX TI - 1st"(w461) -> ()
            n432 = Wait (ms)(milliseconds to wait=u32 500) -> ()  [unwired: 1 out]
          }
        }
        frame #2 {
          n433 = local read "INDEX TI - 1st"() -> (w484:i32)
          n434 = local read "ADDER TI - 1st"() -> (w487:dbl)
          n435 = local read "Array TI - 1st"() -> (w489:dbl[])
          n436 = Increment(x=w484) -> (x+1=w485:i32)
          n437 = Wait (ms)(milliseconds to wait=u32 3000) -> ()  [unwired: 1 out]
          n438 = Insert Into Array(array=w489, index=w485, new element=w487) -> (w488:dbl[])
          n439 = local write "Array TI - 1st"(w488) -> ()
        }
      }
    }
    frame Enabled {
    }
  }
